vi "Main.vi"() -> ()   [LabVIEW 2017]
uses:
  <vilib>/myRIO/Instrument Drivers/Onboard IO/AI/typedefs/AI Reference.ctl
  <vilib>/myRIO/Common/Instrument Driver Framework/Utilities/typedefs/myRIO Generic Hardware Reference.ctl
  <vilib>/myRIO/Common/Instrument Driver Framework/Utilities/typedefs/Hardware Version Enum.ctl
  <vilib>/myRIO/Common/Instrument Driver Framework/Utilities/typedefs/myRIO v1.0 Reference.ctl
  <vilib>/myRIO/Common/Instrument Driver Framework/Utilities/typedefs/Generic FPGA Reference.ctl
  <vilib>/myRIO/Common/Instrument Driver Framework/myRIO v1.0/AI/typedefs/AI Channels List.ctl
  <vilib>/myRIO/Common/Instrument Driver Framework/myRIO v1.0/AI/typedefs/AI Channels Enum.ctl
  <vilib>/myRIO/Common/Instrument Driver Framework/Utilities/typedefs/Analog Scaling Constants List.ctl
  <vilib>/myRIO/Common/Instrument Driver Framework/Utilities/typedefs/Analog Scaling Constants.ctl
  <vilib>/userdefined/High Color/nirio_resource_hc.ctl
  <vilib>/myRIO/Common/Instrument Driver Framework/Utilities/vis/Is FPGA Ref Available.vi
  <vilib>/myRIO/Common/Instrument Driver Framework/myRIO v1.0/AI/vis/myRIO v1.1 Open AI.vi
  <vilib>/myRIO/Instrument Drivers/Onboard IO/AI/vis/Read.vi
  <vilib>/myRIO/Common/Instrument Driver Framework/Utilities/vis/Validate Channels.vi
  <vilib>/myRIO/Common/Instrument Driver Framework/myRIO v1.0/AI/vis/myRIO v1.0 Reserve AI.vi
  <vilib>/myRIO/Common/Instrument Driver Framework/myRIO v1.0/AI/vis/myRIO v1.0 Build MUX Configuration AI.vi
  <vilib>/myRIO/Common/Instrument Driver Framework/myRIO v1.0/Resource Manager/vis/myRIO v1.0 Reserve Channel List.vi
  <vilib>/myRIO/Common/Instrument Driver Framework/myRIO v1.0/Resource Manager/vis/myRIO v1.0 Reserve Channel.vi
  <vilib>/myRIO/Common/Instrument Driver Framework/myRIO v1.0/Resource Manager/vis/myRIO v1.0 Unreserve Channel.vi
  <vilib>/myRIO/Common/Instrument Driver Framework/myRIO v1.0/Resource Manager/vis/myRIO v1.0 Build Mutex Name.vi
  <vilib>/Utility/VariantDataType/GetNumericInfo.vi
  <vilib>/Utility/error.llb/Error Cluster From Error Code.vi
  <vilib>/myRIO/Common/Instrument Driver Framework/myRIO v1.0/myRIO v1.1 Open.vi
  <vilib>/myRIO/Common/Instrument Driver Framework/myRIO v1.0/AI/vis/myRIO v1.0 Get Scaling Constants AI.vi
  <vilib>/myRIO/Common/Instrument Driver Framework/Utilities/vis/IO Manager.vi
  <vilib>/myRIO/Common/Instrument Driver Framework/Utilities/vis/Configuration Manager.vi
  <vilib>/myRIO/Common/Instrument Driver Framework/myRIO v1.0/myRIO v1.0 Close.vi
  <vilib>/myRIO/Common/Instrument Driver Framework/myRIO v1.0/AI/vis/myRIO v1.0 Read AI.vi
  <vilib>/myRIO/Express VI/Onboard IO/AI/AI Express VI.xnode
  <vilib>/myRIO/Instrument Drivers/Onboard IO/AI/vis/myRIO AI Open.xnode
  <vilib>/myRIO/Instrument Drivers/Onboard IO/AI/AI.lvlib
panel:
  out "Output Energy over Time":dbl[](graph)
  out "Output Power over Time":dbl[](graph)
  out "Solar Energy over Time":dbl[](graph)
  out "Solar Power over Time":dbl[](graph)
  out "Total Output Energy (Wh)":dbl
  out "previous output power (W)":dbl
  out "Total Solar Energy (Wh)":dbl
  out "previous solar power (W)":dbl
  out "Full Output":T1
  in  "Load Resistor Value (Ohms)":dbl
  in  "Current Sense Resistor Value (Ohms)":dbl
  out "ADC Readings (rounded)":T2
  in  "Rouding Factor":T3(ring)
  in  "milliseconds to wait":u32(slide)=100 max=1000 step=100 scale=0.0..1000.0
  in  "stop":bool
  # "These are for internal use only"
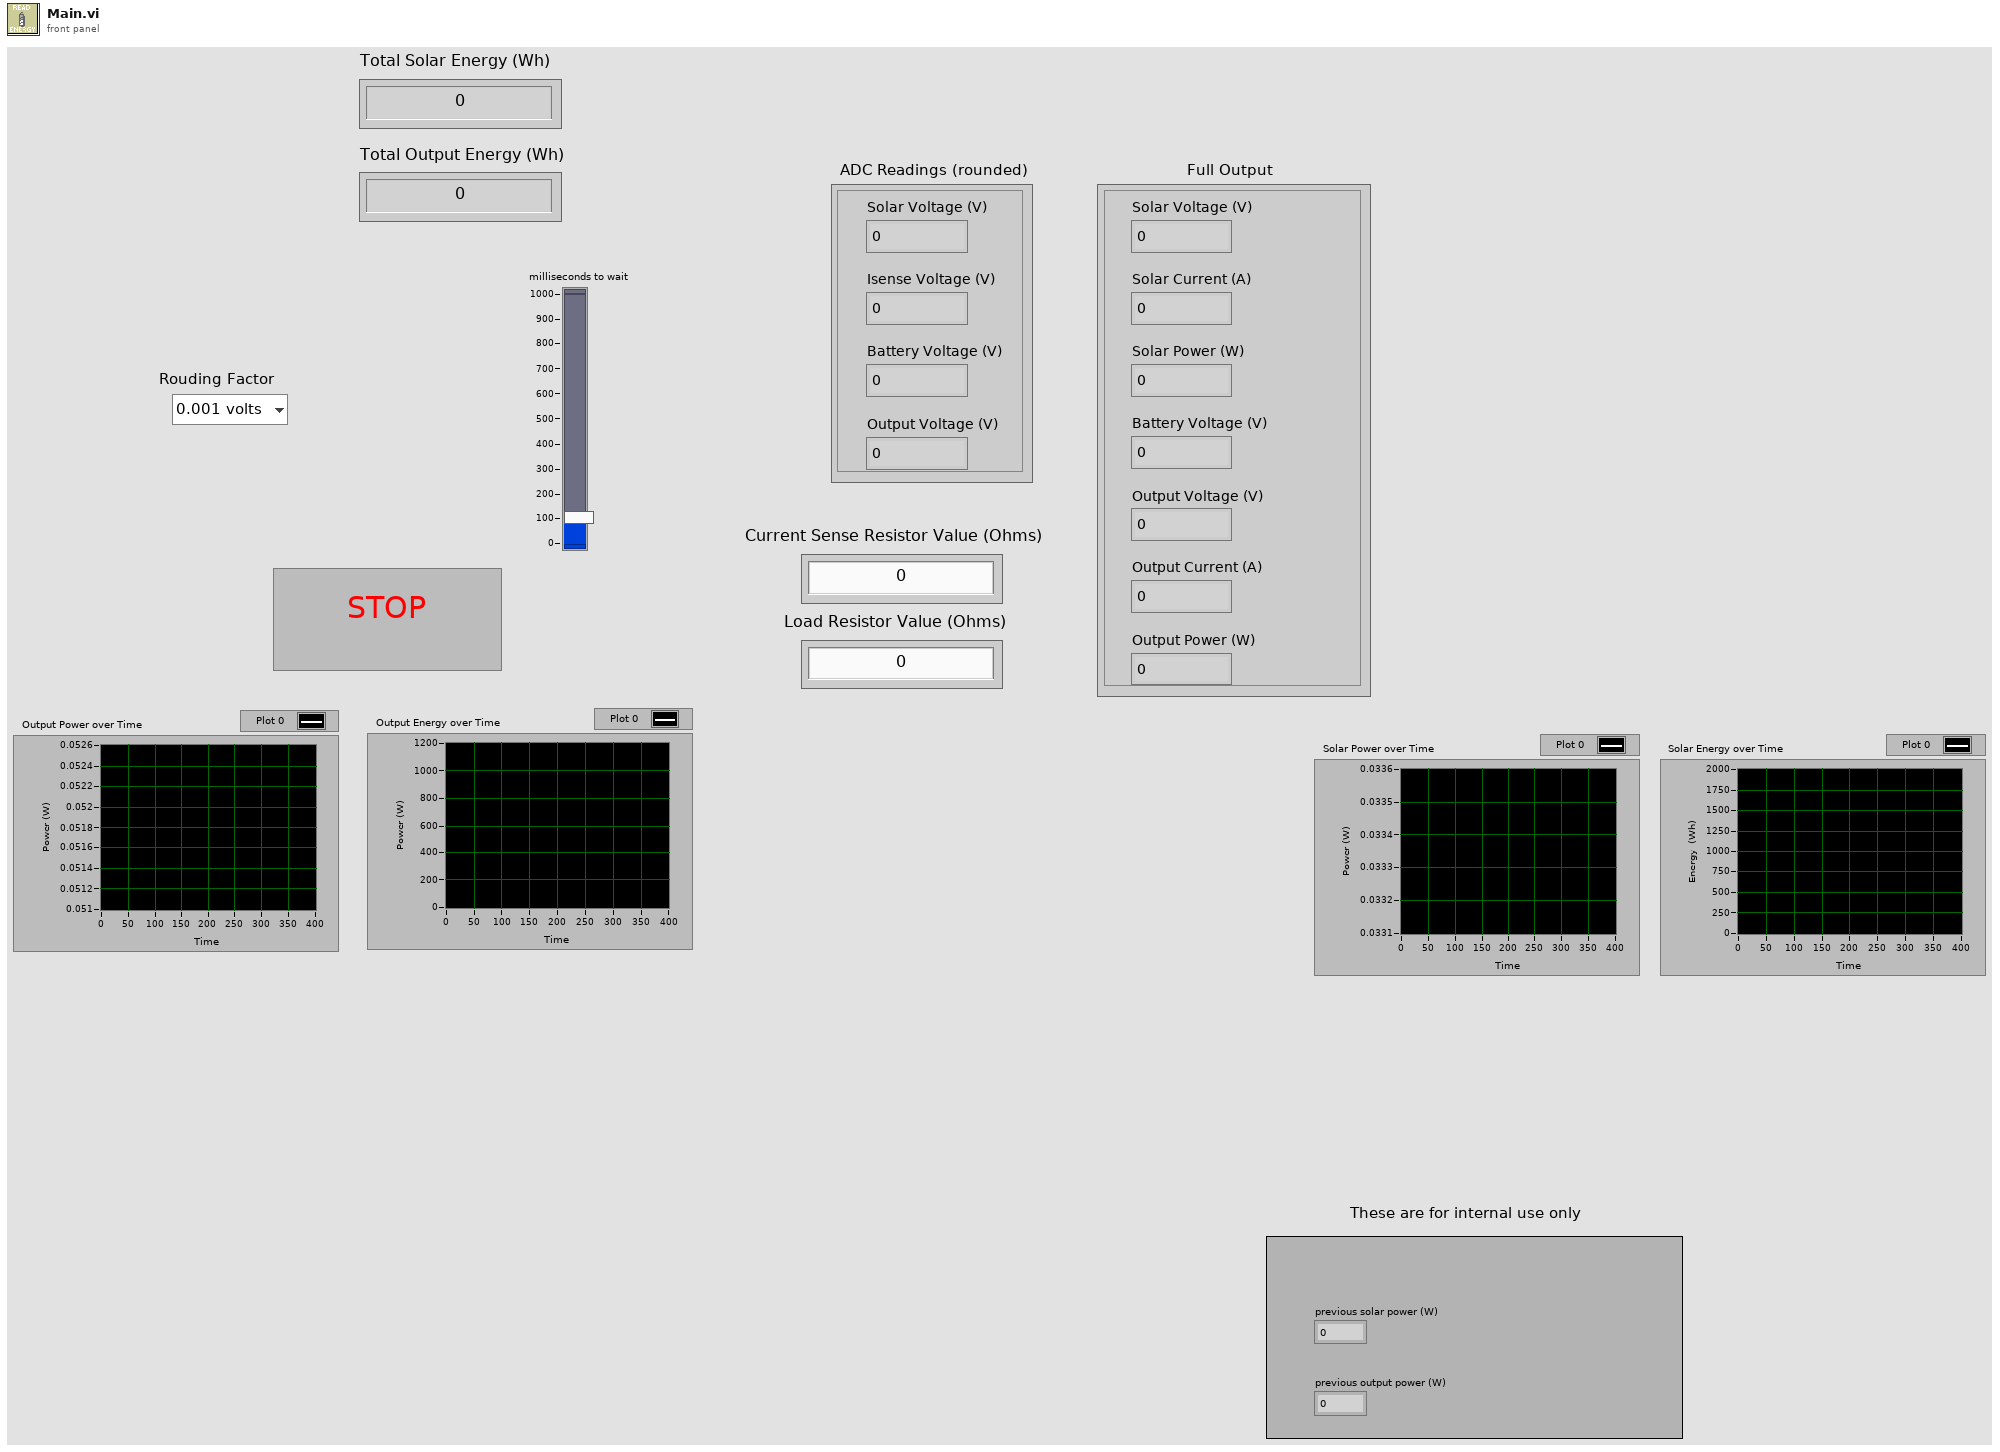
[diagram p1: front panel]
types:
  T1 = cluster{"Solar Voltage (V)":dbl, "Solar Current (A)":dbl, "Solar Power (W)":dbl, "Battery Voltage (V)":dbl, "Output Voltage (V)":dbl, "Output Current (A)":dbl, "Output Power (W)":dbl}
  T2 = cluster{"Solar Voltage (V)":dbl, "Isense Voltage (V)":dbl, "Battery Voltage (V)":dbl, "Output Voltage (V)":dbl}
  T3 = enum16{"0.001 volts", "0.01 volts", "0.1 volts", "1 volt"}
  T4 = typedef "AI.lvlib/AI Reference.ctl" = cluster{"myRIO Reference":T5, "AI Channels List":T9, "AI Scaling Constants List":T11}
  T5 = typedef "myRIO Generic Hardware Reference.ctl" = cluster{"myRIO Model":T6, "myRIO Hardware Reference":T7}
  T6 = typedef "Hardware Version Enum.ctl" = enum16{"Unknown", "myRIO-1900", "myRIO-1950", "roboRIO", "NI ELVIS RIO CM"}
  T7 = typedef "myRIO v1.0 Reference.ctl" = cluster{"Generic FPGA Reference":T8, "Allow multiple opens":bool}
  T8 = typedef "Generic FPGA Reference.ctl" = refnum<k20>
  T9 = typedef "AI Channels List.ctl" = T10[]
  T10 = typedef "AI Channels Enum.ctl" = enum16{"Not Connected", "AudioIn/Left", "AudioIn/Right", "C/AI0", "C/AI1", "A/AI0", "A/AI1", "A/AI2", "A/AI3", "B/AI0", "B/AI1", "B/AI2", "B/AI3", "AI/AI0", "AI/AI1", "AI/AI2", "AI/AI3"}
  T11 = typedef "Analog Scaling Constants List.ctl" = T12[]
  T12 = typedef "Analog Scaling Constants.ctl" = cluster{"LSB Weight (Volts)":dbl, "Offset (Volts)":dbl, "Signed?":bool}
  T13 = typedef "nirio_resource_hc.ctl" = tag
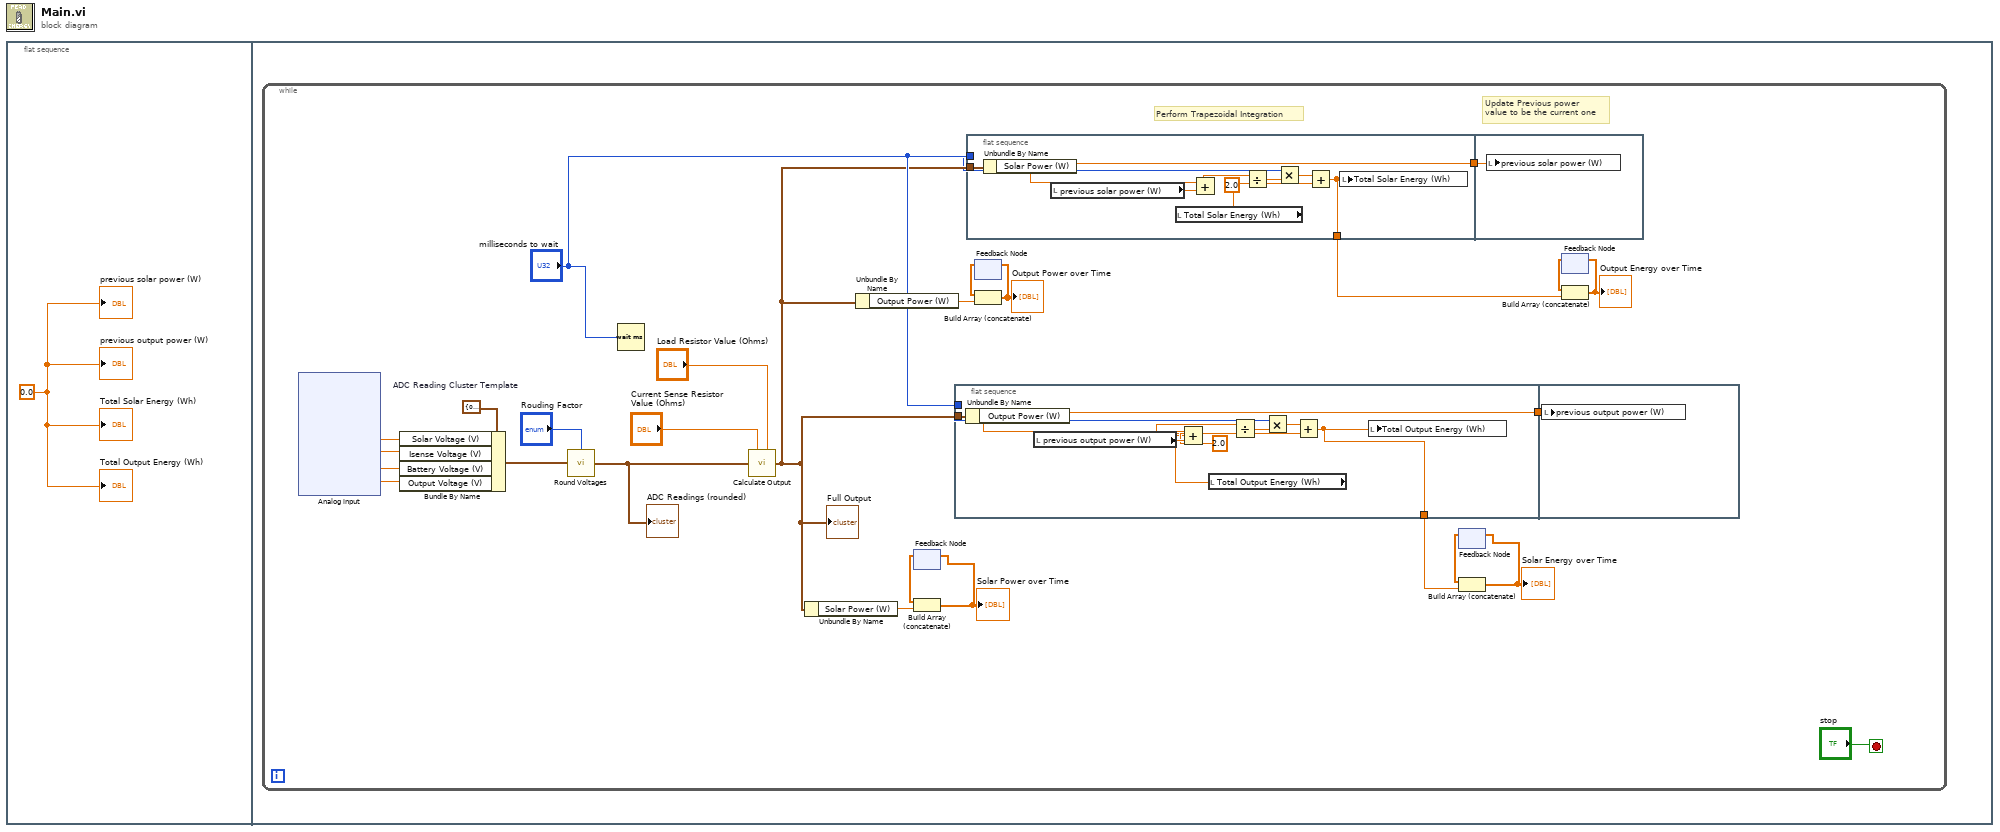
[diagram p0: block diagram]
diagram:
  n1 = flat-sequence {
    frame #0 {
      w1 = 0.0 ("Total Solar Energy (Wh)")
      "previous solar power (W)" <- w1
      "Total Solar Energy (Wh)" <- w1
      "previous output power (W)" <- w1
      "Total Output Energy (Wh)" <- w1
    }
    frame #1 {
      n2 = while {
        stop <- "stop" stop-if-true
        w22 = T2 {"Solar Voltage (V)"=0.0, "Isense Voltage (V)"=0.0, "Battery Voltage (V)"=0.0, "Output Voltage (V)"=0.0}  # ADC Reading Cluster Template
        # "Update Previous power\nvalue to be the current one"
        # "Perform Trapezoidal Integration"
        n3 = xnode "Analog input"() -> ("Solar Voltage (A/AI0 (Pin 3))"=w27:dbl, "Isense Voltage (A/AI1 (Pin 5))"=w26:dbl, "Battery Voltage (A/AI2 (Pin 7))"=w25:dbl, "Output Voltage (A/AI3 (Pin 9))"=w24:dbl)  [unwired: 1 in, 1 out]
        n4 = Bundle By Name(cluster=w22, "Solar Voltage (V)"=w27, "Isense Voltage (V)"=w26, "Battery Voltage (V)"=w25, "Output Voltage (V)"=w24) -> (w21:T2)
        n5 = call "Round Voltages.vi"("Rouding Factor (0.001 volts)"="Rouding Factor", "ADC Readings (input)"=w21) -> ("ADC Readings (rounded)"=w20:T2)  [unwired: 13 in]
        "ADC Readings (rounded)" <- w20
        n6 = Wait (ms)(milliseconds to wait="milliseconds to wait") -> ()  [unwired: 1 out]
        n7 = call "Calculate Output.vi"("Current Sense Resistor Value (Ohms)"="Current Sense Resistor Value (Ohms)", "Load Resistor Value (Ohms)"="Load Resistor Value (Ohms)", "ADC Readings (input)"=w20) -> ("Full Output"=w8:T1)  [unwired: 12 in]
        "Full Output" <- w8
        n8 = Unbundle By Name(w8) -> ("Solar Power (W)"=w9:dbl)
        n9 = Unbundle By Name(w8) -> ("Output Power (W)"=w7:dbl)
        n10 = feedback #1() -> (w10:dbl[])  [unwired: 1 in]
        n11 = Build Array (concatenate) "Build Array"(w10, w9) -> (w14:dbl[])
        "Solar Power over Time" <- w14
        n12 = feedback-in #1(w14) -> ()
        n13 = flat-sequence {
          tunnel: w8 -> [w38]
          tunnel: "milliseconds to wait" -> [w33]
          tunnel: [w31] -> w16
          tunnel: [w29] -> w11
          tunnel: w16 -> [w39]
          frame #0 {
            n14 = Unbundle By Name(w38) -> ("Output Power (W)"=w31:dbl)
            n15 = local read "previous output power (W)"() -> (w37:dbl)
            n16 = Add(x=w31, y=w37) -> (x+y=w35:dbl)
            n17 = local read "Total Output Energy (Wh)"() -> (w30:dbl)
            n18 = Divide(x=w35, y=2.0) -> (x/y=w34:dbl)
            n19 = Multiply(x=w33, y=w34) -> (x*y=w32:dbl)
            n20 = Add(x=w32, y=w30) -> (x+y=w29:dbl)
            n21 = local write "Total Output Energy (Wh)"(w29) -> ()
          }
          frame #1 {
            n22 = local write "previous output power (W)"(w39) -> ()
          }
        }
        n23 = flat-sequence {
          tunnel: w8 -> [w48]
          tunnel: "milliseconds to wait" -> [w43]
          tunnel: [w41] -> w17
          tunnel: [w40] -> w2
          tunnel: w17 -> [w50]
          frame #0 {
            n24 = Unbundle By Name(w48) -> ("Solar Power (W)"=w41:dbl)
            n25 = local read "previous solar power (W)"() -> (w47:dbl)
            n26 = local read "Total Solar Energy (Wh)"() -> (w49:dbl)
            n27 = Add(x=w41, y=w47) -> (x+y=w45:dbl)
            n28 = Divide(x=w45, y=2.0) -> (x/y=w44:dbl)
            n29 = Multiply(x=w43, y=w44) -> (x*y=w42:dbl)
            n30 = Add(x=w42, y=w49) -> (x+y=w40:dbl)
            n31 = local write "Total Solar Energy (Wh)"(w40) -> ()
          }
          frame #1 {
            n32 = local write "previous solar power (W)"(w50) -> ()
          }
        }
        n33 = feedback #2() -> (w6:dbl[])  [unwired: 1 in]
        n34 = Build Array (concatenate)(w6, w7) -> (w5:dbl[])
        "Output Power over Time" <- w5
        n35 = feedback-in #2(w5) -> ()
        n36 = feedback #3() -> (w12:dbl[])  [unwired: 1 in]
        n37 = Build Array (concatenate) "Build Array"(w12, w11) -> (w13:dbl[])
        "Solar Energy over Time" <- w13
        n38 = feedback-in #3(w13) -> ()
        n39 = feedback #4() -> (w3:dbl[])  [unwired: 1 in]
        n40 = Build Array (concatenate)(w3, w2) -> (w4:dbl[])
        "Output Energy over Time" <- w4
        n41 = feedback-in #4(w4) -> ()
      }
    }
  }
